vi "LEBITVacuum.ProcConstructor.vi"(0 "i ref in":refnum<vi>, 5 "error in(no error)":errorcluster) -> (14 "i ref out":refnum<vi>, 19 "error out":errorcluster)   [LabVIEW 2014, in "LEBITVacuum.lvlib"]
doc: "This is the constructor of a class.\n\nLicense Agreement for this software:\n\nCopyright (C)\nGesellschaft für Schwerionenforschung, GSI\nPlanckstr. 1\n64291 Darmstadt\nGermany\n\nContact: D.Beck@gsi.de \n\nThis program is free software; you can redistribute it and/or modify it under the terms of the \nGNU General Public License as published by the Free Software Foundation; either version 2 of \nthe license, or (at your option) any later version.\n\nThis program is distributed in the hope that it will be useful, but WITHOUT ANY WARRANTY; \nwithout even the implied warranty of MERCHANTABILITY or FITNESS FOR A PARTICULAR PURPOSE. See the GNU General License for more details (http://www.gnu.org).\n\nGesellschaft für Schwerionenforschung, GSI\nPlanckstr. 1, 64291 Darmstadt, Germany\nFor all questions and ideas contact: M.Richter@gsi.de, H.Brand@gsi.de or D.Beck@gsi.de.\nLast update: 16-JUN-2004"
uses:
  LEBITVacuum.lvlib
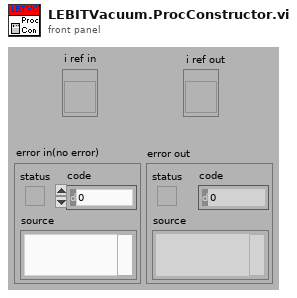
[diagram p1: front panel]
types:
  T1 = typedef "LEBITVacuum.lvlib/LEBITVacuum.i attribute.ctl" = cluster{"setValuePLC":string[], "nickNames":string[], "setValuePLCServiceID":i32[], "monValuePLC":string[], "SetValueServiceID":i32[], "MonValueServiceID":i32[], "SetValue":i16[], "AllPLCValues":string[], "CondSpecial2DArray":string[][], "CondSpecialIndex":i32[], "ReasonForLocking":string, "ReasonForLockingID":i32, "enableValuePLC":string[], "OverwriteCloseSafetyPLC":string[], "OverwriteOpenSafetyPLC":string[], "OverwriteCloseSafetyPLCServiceID":i32[], "OverwriteOpenSafetyPLCServiceID":i32[], "MKS Address Array":i32[][], "MKS MeasurementServiceID":i32[], "MKS Measurement":string[], "CRYO Measurement":string[][], "CRYO MeasurementServiceID":i32[], "Special":string[], "Start Date":string, "MKS VISA resource":refnum<visa-resource-name>, "CRYO VISA resource":refnum<visa-resource-name>}
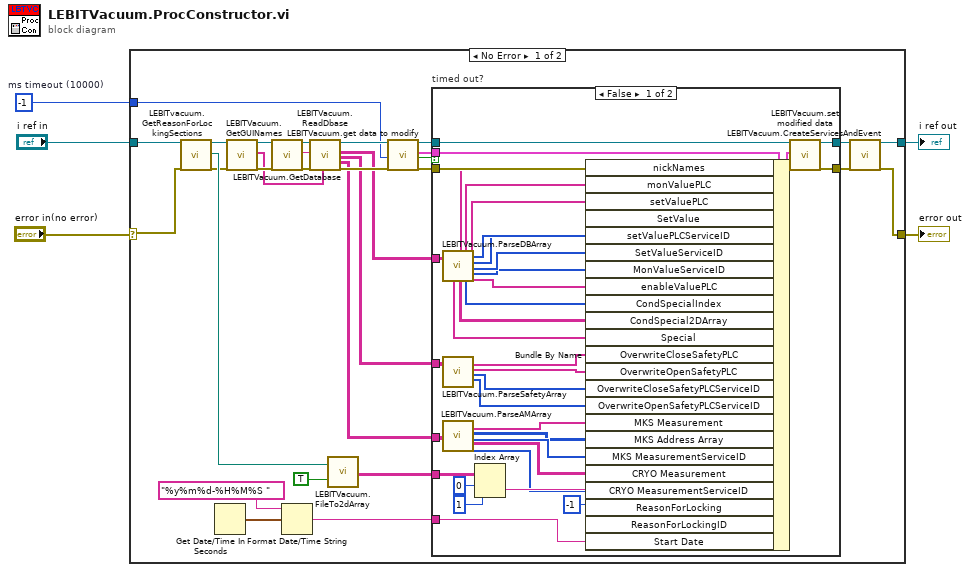
[diagram p0: block diagram]
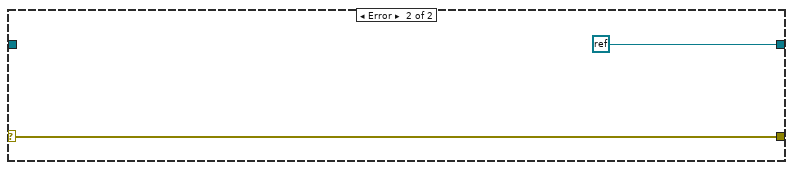
[diagram p3: hidden frame]
diagram:
  w1 = -1  # ms timeout (10000)
  n1 = case shown="No Error" "error in(no error)" {
    selector: "error in(no error)" -> [w19 w74]
    tunnel: [w21 w74] -> w5
    tunnel: "i ref in" -> [w20 _]
    tunnel: [w22 refnum<k0> refnum] -> w2
    tunnel: w1 -> [w25 _]
    frame No Error {
      n2 = call "LEBITvacuum.GetReasonForLockingSections.vi"("i ref in"=w20, "error in (no error)"=w19) -> ("i ref out"=w13:refnum<vi>, "Last Loaded File Loaction"=w16:path, "error out"=w12:errorcluster)  [unwired: 15 in]
      n3 = Get Date/Time In Seconds() -> (seconds since 1Jan1904=w8:timestamp)
      n4 = call "LEBITVacuum.GetGUINames.vi"("i ref in"=w13, "error in (no error)"=w12) -> ("i ref out"=w11:refnum<vi>, "GUINames"=w9:string[], "error out"=w10:errorcluster)  [unwired: 15 in]
      n5 = call "LEBITVacuum.GetDatabase.vi"("i ref in"=w11, "error in (no error)"=w10) -> ("i ref out"=w31:refnum<vi>, "database"=w33:string, "error out 2"=w34:errorcluster)  [unwired: 15 in]
      n6 = Format Date/Time String(time format string (%c)="%y%m%d-%H%M%S ", seconds (now)=w8) -> (date/time string=w7:string)  [unwired: 1 in]
      n7 = call "LEBITVacuum.ReadDbase.vi"("i ref in"=w31, "Data Source"=w33, "error in (no error)"=w34, "Associated Panels"=w9) -> ("i ref out"=w30:refnum<vi>, "DBArray"=w26:string[][], "Safety Array"=w18:string[][], "Ambient Measurements"=w17:string[][], "error out"=w32:errorcluster)  [unwired: 11 in]
      n8 = call "LEBITVacuum.FileTo2dArray.vi"("file path (dialog if empty)"=w16, "Create if ness."=TRUE) -> ("Array"=w15:string[][])  [unwired: 16 in, 1 out]
      n9 = call "LEBITVacuum.get data to modify.vi"("i ref in"=w30, "ms timeout (10000)"=w25, "error in (no error)"=w32) -> ("i ref out"=w28:refnum<vi>, "i attribute"=w35:T1, "timed out"=w29:bool, "error out"=w27:errorcluster)  [unwired: 13 in]
      n10 = case "timed out?" shown="False" w29 {
        tunnel: w35 -> [w66 _]
        tunnel: w28 -> [w68 w72]
        tunnel: [w70 w72] -> w24
        tunnel: [w69 w71] -> w23
        tunnel: w27 -> [w62 w71]
        tunnel: w26 -> [w67 _]
        tunnel: w15 -> [w50 _]
        tunnel: w18 -> [w49 _]
        tunnel: w17 -> [w45 _]
        tunnel: w7 -> [w36 _]
        frame False {
          n11 = call "LEBITVacuum.ParseDBArray.vi"("DBArray"=w67) -> ("Special"=w37:string[], "nickname"=w61:string[], "CondSpecial2DArray"=w51:string[][], "monValuePLC"=w65:string[], "SpecialIndex"=w52:i32[], "setValuePLC"=w64:string[], "SetValue"=w57:i16[], "setValuePLCServiceID"=w56:i32[], "SetValueServiceID"=w55:i32[], "MonValueServiceID"=w54:i32[], "enableValuePLC"=w53:string[])  [unwired: 8 in]
          n12 = call "LEBITVacuum.ParseSafetyArray.vi"("Safety Array"=w49) -> ("CloseSafetyOverwritePLC"=w38:string[], "OpenSafetyOverwritePLC"=w48:string[], "CloseSafetyOverwritePLCServiceID"=w47:i32[], "OpenSafetyOverwritePLCServiceID"=w46:i32[])  [unwired: 15 in]
          n13 = call "LEBITVacuum.ParseAMArray.vi"("AMArray"=w45) -> ("MKS Measurement"=w44:string[], "MKS Address Array"=w39:i32[][], "MKS MeasurementServiceID"=w43:i32[], "CRYO Measurement"=w41:string[][], "CRYO MeasurementServiceID"=w40:i32[])  [unwired: 14 in]
          n14 = Index Array(array=w50, index (row)=0, index (col)=1 ("disabled index (col)")) -> (element=w42:string)
          n15 = Bundle By Name(cluster=w66, "nickNames"=w61, "monValuePLC"=w65, "setValuePLC"=w64, "SetValue"=w57, "setValuePLCServiceID"=w56, "SetValueServiceID"=w55, "MonValueServiceID"=w54, "enableValuePLC"=w53, "CondSpecialIndex"=w52, "CondSpecial2DArray"=w51, "Special"=w37, "OverwriteCloseSafetyPLC"=w38, "OverwriteOpenSafetyPLC"=w48, "OverwriteCloseSafetyPLCServiceID"=w47, "OverwriteOpenSafetyPLCServiceID"=w46, "MKS Measurement"=w44, "MKS Address Array"=w39, "MKS MeasurementServiceID"=w43, "CRYO Measurement"=w41, "CRYO MeasurementServiceID"=w40, "ReasonForLocking"=w42, "ReasonForLockingID"=-1, "Start Date"=w36) -> (w63:T1)
          n16 = call "LEBITVacuum.set modified data.vi"("i ref in"=w68, "i attribute"=w63, "error in (no error)"=w62) -> ("i ref out"=w70:refnum<vi>, "error out"=w69:errorcluster)  [unwired: 15 in]
        }
        frame True {
        }
      }
      n17 = call "LEBITVacuum.CreateServicesAndEvent.vi"("i ref in"=w24, "error in(no error)"=w23) -> ("i ref out"=w22:refnum<vi>, "error out"=w21:errorcluster)  [unwired: 16 in]
    }
    frame Error {
    }
  }
  "i ref out" <- w2
  "error out" <- w5
